vi "GV_Repos.vi"() -> ()   [LabVIEW 2016, in "WSsupport.lvlib"]
uses:
  Packages/Repo_class/Repo.lvclass
  WSsupport.lvlib
panel:
  in  "Repos":refnum<class "Repo.lvclass">[](array[class])
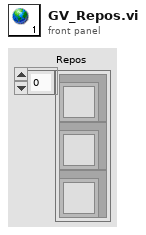
[diagram p1: front panel]
diagram:
